vi "SEK2020v1SubVIComparaCor.vi"(6 "Branco Min EV3 Cor":sgl, 9 "Branco Max EV3 Cor":sgl, 10 "Scaled Value 2":sgl, 11 "Scaled Value":sgl) -> (3 "Boolean":bool)   [LabVIEW 2016]
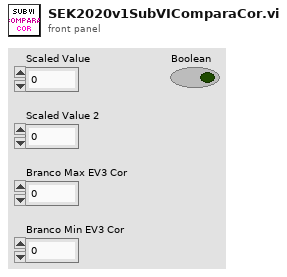
[diagram p1: front panel]
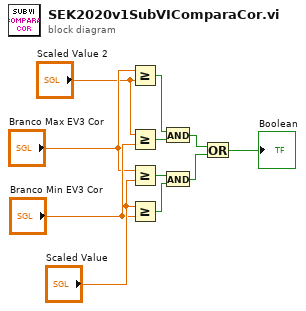
[diagram p0: block diagram]
diagram:
  n1 = Greater Or Equal?(x="Branco Max EV3 Cor", y="Scaled Value 2") -> (x >= y?=w5:bool)
  n2 = Greater Or Equal?(x="Scaled Value 2", y="Branco Min EV3 Cor") -> (x >= y?=w4:bool)
  n3 = Greater Or Equal?(x="Branco Max EV3 Cor", y="Scaled Value") -> (x >= y?=w10:bool)
  n4 = Greater Or Equal?(x="Scaled Value", y="Branco Min EV3 Cor") -> (x >= y?=w11:bool)
  n5 = And(x=w5, y=w4) -> (x .and. y?=w2:bool)
  n6 = And(x=w10, y=w11) -> (x .and. y?=w3:bool)
  n7 = Or(x=w2, y=w3) -> (x .or. y?=→"Boolean":bool)
